vi "TEST_ASIC_MAJ_NEW.vi"(7 "Serial Number":string="SN_1234", 8 "error in":errorcluster, 11 "Instrument VISA in":T1={"AWG VISA"="AgilentGenerator1", "Oscilloscope  VISA "="AgilentOsciloscope", "Integration Board IP"="172.16.17.47", "connection ID"=refnum, "report out"=refnum, "report file path"=path "C:/Users/omartinez/Desktop/L0nL1_Results"}) -> (0 "error out":errorcluster, 3 "Instrument VISA out":T1={"AWG VISA"="AgilentGenerator1", "Oscilloscope  VISA "="AgilentOsciloscope", "Integration Board IP"="172.16.17.47", "connection ID"=refnum, "report out"=refnum, "report file path"=path "C:/Users/omartinez/Desktop/L0nL1_Results"}, 5 "ThresholdOut":i32[][](array[numeric])=[[526, 520, 522, 524, 510, 512, 524]])   [LabVIEW 2012]
uses:
  <vilib>/Utility/NIReport.llb/NI_report.lvclass
  <vilib>/Utility/NIReport.llb/HTML/NI_HTML.lvclass
  <instrlib>/Agilent 8000 Series/Public/Configure/Configure Math (Binary Operation).vi
  Sum_Abrilader/L0_Sum_Adder Folder/C/Program Files/National Instruments/LabVIEW 2012/instr.lib/Agilent 8000 Series/Public/Data/Low Level/Fetch Measurement (More).vi
  <instrlib>/Agilent 8000 Series/Agilent 8000 Series.lvlib
  Sum_Abrilader/L0_Sum_Adder Folder/C/Program Files/National Instruments/LabVIEW 2012/instr.lib/Agilent 81150/Agilent 81150.lvlib
panel:
  in  "Clip_sel_b":u32=1
  in  "Ib_clipVb":u32=63
  in  "Att gain":u32=15
  out "threshold out":i32=524
  in  "Threshold Limits":i32[](array[numeric])=[500, 1024]
  in  "Channels":i32[](array[numeric])=[0, 1, 2, 3, 4, 5, 6]
  in  "Voltages comprobation":dbl[](array[numeric])=[0.05, 0.1, 0.2, 0.5, 0.8]
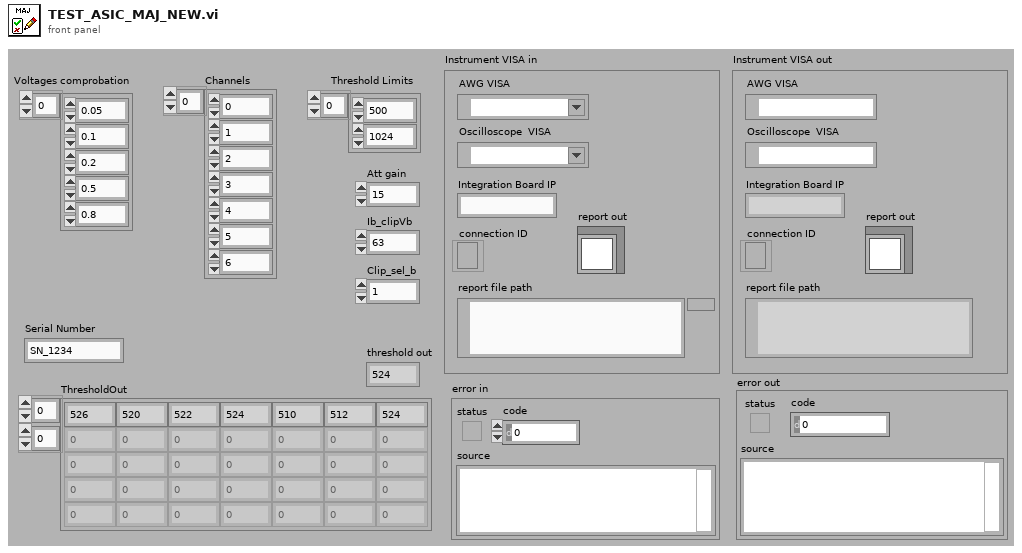
[diagram p1: front panel]
types:
  T1 = cluster{"AWG VISA":refnum<visa-resource-name>, "Oscilloscope  VISA ":refnum<visa-resource-name>, "Integration Board IP":string, "connection ID":refnum<k5>, "report out":refnum<class "NI_report.lvclass">, "report file path":path}
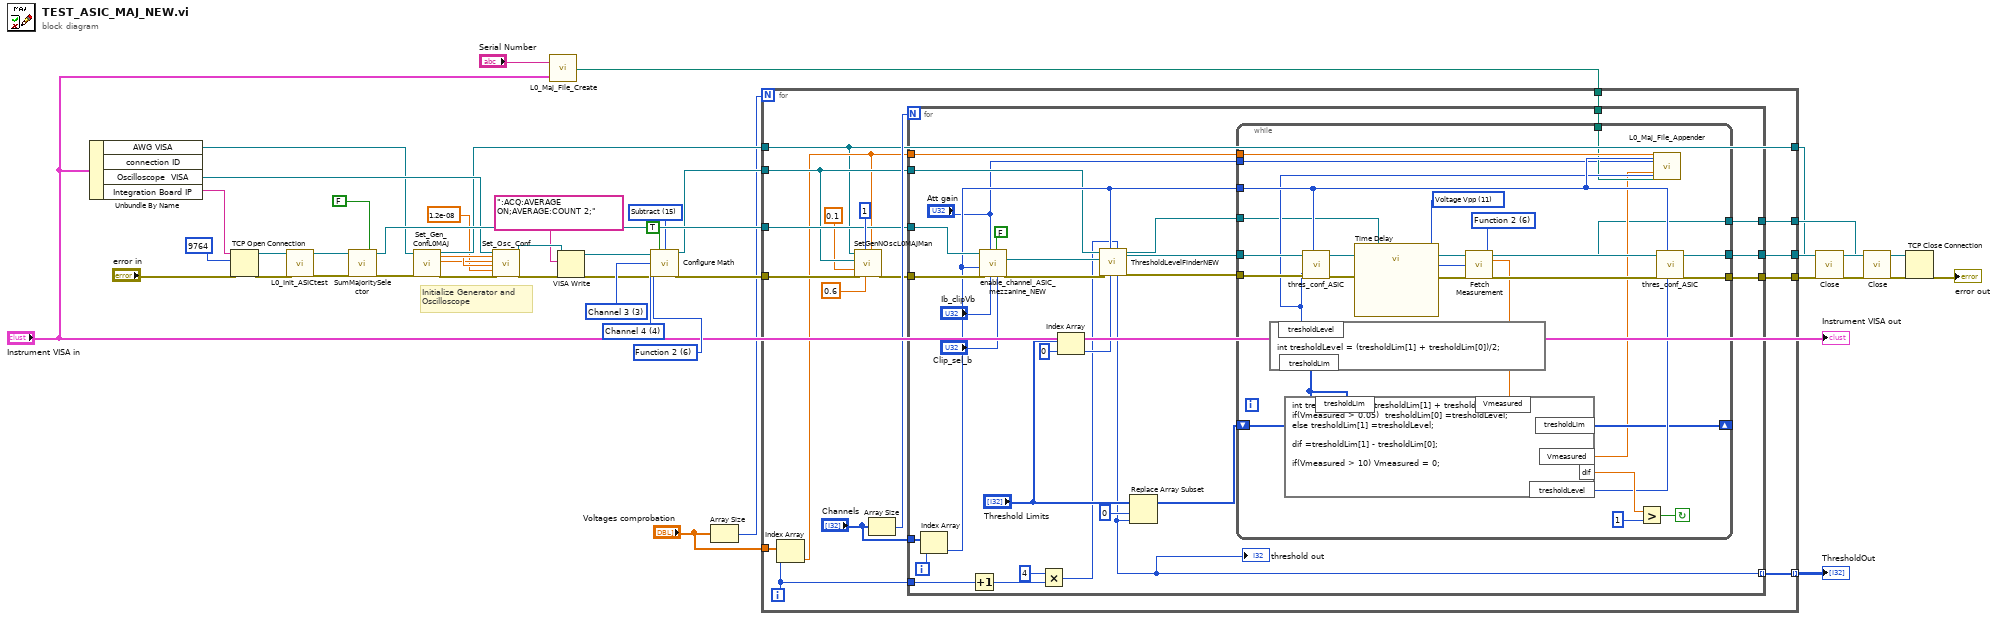
[diagram p0: block diagram]
diagram:
  w30 = u16 6 items=["Function 1"=5, "Function 2"=6, "Function 3"=7, "Function 4"=8] ("Math Channel (5: Function 1)")
  w31 = u16 15 items=["Add"=12, "Divide"=13, "Multiply"=14, "Subtract"=15, "Common Mode"=16, "Versus"=17] ("Math Operation (12: Add)")
  w29 = 3 items=["Channel 1"=1, "Channel 2"=2, "Channel 3"=3, "Channel 4"=4] ("Channel (1: Channel 1)")
  w28 = 4 items=["Channel 1"=1, "Channel 2"=2, "Channel 3"=3, "Channel 4"=4] ("Channel (1: Channel 1)")
  # "Initialize Generator and \nOscilloscope"
  n1 = Unbundle By Name("Instrument VISA in") -> ("AWG VISA"=w7:refnum<visa-resource-name>, "Oscilloscope  VISA"=w11:refnum<visa-resource-name>, "Integration Board IP"=w40:string)  [unwired: 1 out]
  n2 = TCP Open Connection(address=w40, remote port or service name=u16 9764, error in (no error)="error in") -> (connection ID=w34:refnum<k5>, error out=w35:errorcluster)  [unwired: 2 in]
  n3 = call "L0_Init_ASICtest.vi"("error in"=w35, "connection ID in"=w34) -> ("error out"=w36:errorcluster, "connection ID out"=w33:refnum<k5>)  [unwired: 8 in]
  n4 = call "SumMajoritySelector.vi"("On Sum\nOff Majority"=FALSE ("On Sum\nOff Majority"), "error in (no error)"=w36, "connection ID"=w33) -> ("error out"=w8:errorcluster, "connection ID out"=w39:refnum<k5>)  [unwired: 5 in]
  n5 = call "Set_Gen_ConfL0MAJ.vi"("AWG VISA"=w7, "error in (no error)"=w8) -> ("Amplitude 1 OUT"=w16:dbl, "VISA resource name out"=w6:refnum<visa-resource-name>, "Pulse Width in seconds 1 OUT"=w15:dbl, "Trigger Level 1"=w14:dbl, "error out"=w17:errorcluster)  [unwired: 10 in, 3 out]
  n6 = call "Set_Osc_Conf.vi"("VISA resource name"=w11, "Amplitude IN"=w16, "Trigger Level IN"=w14, "Pulse Width in seconds IN"=w15, "Position 1"=1.2e-08, "error in (no error)"=w17) -> ("VISA resource name out"=w12:refnum<visa-resource-name>, "error out"=w13:errorcluster)  [unwired: 12 in]
  n7 = call "L0_Maj_File_Create.vi"("input cluster"="Instrument VISA in", "Serial Number"="Serial Number") -> ("appended path"=w21:path)
  n8 = VISA Write(VISA resource name=w12, write buffer=":ACQ:AVERAGE ON;AVERAGE:COUNT 2;", error in (no error)=w13) -> (VISA resource name out=w10:refnum<visa-resource-name>, error out=w9:errorcluster)  [unwired: 1 out]
  n9 = call-poly <instrlib>:"Configure Math.vi"("VISA resource name"=w10, "Enable Math Channel (T:Enable)"=TRUE, "Math Operation (12: Add)"=w31, "Math Channel (5: Function 1)"=w30, "Math Operand (1: Channel 1)"=w29, "Math Operand (2: Channel 2)"=w28, "error in (no error)"=w9) -> ("VISA resource name out"=w26:refnum<visa-resource-name>, "error out"=w27:errorcluster)  [unwired: 7 in]
  n10 = Array Size(array="Voltages comprobation") -> (size(s)=w1:i32)
  n11 = for {
    N: w1 -> [_]
    tunnel: [w61] -> w19
    tunnel: [w60] -> w41
    tunnel: w27 -> [w56]
    tunnel: w39 -> [w52]
    tunnel: w6 -> [w44]
    tunnel: w26 -> [w51]
    tunnel: "Voltages comprobation" -> [w59]
    tunnel: [w50] -> w24 mode=indexing
    tunnel: w21 -> [w49]
    tunnel: [w45] -> w5
    tunnel: [w44] -> w4
    i -> [w46]
    n12 = Index Array(array=w59, index=w46) -> (element=w47:dbl)
    n13 = call "SetGenNOscL0MAJMan.vi"("Input Voltage"=w47, "Amp Scaler"=0.6, "NChannels"=1, "error in (no error)"=w56, "Output Voltage"=0.1 ("Input Voltage"), "VISA resource name"=w51, "AWG VISA"=w44) -> ("error out 2"=w53:errorcluster)  [unwired: 4 in]
    n14 = Array Size(array="Channels") -> (size(s)=w54:i32)
    n15 = for {
      N: w54 -> [_]
      tunnel: [w90] -> w61
      tunnel: [w89] -> w60
      tunnel: "Channels" -> [w87]
      tunnel: w53 -> [w86]
      tunnel: w52 -> [w82]
      tunnel: w51 -> [w79]
      tunnel: w47 -> [w74]
      tunnel: [w64] -> w50 mode=indexing
      tunnel: w49 -> [w72]
      tunnel: w46 -> [w68]
      tunnel: [w66] -> w45
      i -> [w88]
      n16 = Index Array(array=w87, index=w88) -> (element=w81:i32)
      n17 = Increment(x=w68) -> (x+1=w65:i32)
      n18 = call "enable_channel_ASIC_mezzanine_NEW.vi"("Clip_sel_b"="Clip_sel_b", "maj/sum"=FALSE, "Ib_clipVb"="Ib_clipVb", "Att gain"="Att gain", "error in"=w86, "Channel"=w81, "connection ID"=w82) -> ("error out"=w80:errorcluster, "connection ID out"=w78:refnum<k5>)  [unwired: 2 in, 1 out]
      n19 = Multiply(x=4, y=w65) -> (x*y=w63:i32)
      n20 = Index Array(array="Threshold Limits", index=0) -> (element=w77:i32)
      n21 = call "ThresholdLevelFinderNEW.vi"("correction"=w63, "Initial Threshold"=w77, "Channel"=w81, "error in (no error)"=w80, "connection ID"=w78, "VISA resource name"=w79) -> ("error out"=w62:errorcluster, "connection ID out"=w75:refnum<k5>, "VISA resource name out"=w73:refnum<visa-resource-name>, "threshold out"=w64:i32)  [unwired: 1 in, 1 out]
      "threshold out" <- w64
      n22 = Replace Array Subset(array="Threshold Limits", new element=w64, index=u32 0 ("Att gain")) -> (w76:i32[])
      n23 = while {
        tunnel: [w105] -> w90
        tunnel: [w104] -> w89
        tunnel: w81 -> [w102]
        tunnel: w75 -> [w116]
        tunnel: w62 -> [w115]
        shift-right: [w98] -> _
        shift-left: w76 -> [w111]
        tunnel: w74 -> [w103]
        tunnel: w73 -> [w99]
        tunnel: w72 -> [w97]
        tunnel: "Att gain" -> [w94]
        tunnel: [w93] -> w66
        stop <- w112 continue-if-true
        w109 = 11 items=["Rise Time", "Fall Time", "Frequency", "Period", "Voltage RMS(AC)", "Voltage RMS(DC)", "Voltage RMS (AC,cycle)", "Voltage RMS (DC,cycle)", "Voltage Max", "Voltage Min", "Voltage Middle", "Voltage Vpp", "Voltage High", "Voltage Low", "Voltage Average", "Voltage Average (cycle)", "Width Negative", "Width Positive", "Duty Cycle Positive", "Amplitude", "Overshoot", "Preshoot", "Voltage Base", "Voltage Upper", "Time Max", "Time Min", "Color Grade Crossing", "Color Grade Eye Width", "Color Grade Eye Height", "Color Grade Eye Q-Factory", "Color Grade Eye Duty Cycle Distortion(Percent)", "Color Grade Eye Duty Cycle Distortion(Time)", "Color Grade Eye Jitter(PP)", "Color Grade Eye Width(RMS)", "Cycle-cycle Duty Jitter(Rising)", "Cycle-cycle Duty Jitter(Falling)", "Cycle-cycle Jitter(Rising)", "Cycle-cycle Jitter(Falling)", "Cycle-cycle - Width", "Cycle-cycle + Width", "Date Rate", "Unit Interval", "FFT Delta Frequency", "FFT Delta Magnitude", "FFT Frequency", "FFT Magnitude", "Slew Rate", "Area (Entire Display)", "Area(Single Cycle)", "Duty Cycle (Rising)", "Duty Cycle (Falling)"] ("Measurement Function (0: Rise Time)")
        w110 = 6 items=["Channel 1"=1, "Channel 2"=2, "Channel 3"=3, "Channel 4"=4, "Function 1"=5, "Function 2"=6, "Function 3"=7, "Function 4"=8, "Memory 1"=9, "Memory 2"=10, "Memory 3"=11, "Memory 4"=12] ("Channel (1: Channel 1)")
        n24 = formula code="int tresholdLevel = (tresholdLim[1] + tresholdLim[0])/2;"("tresholdLim"=w111) -> ("tresholdLevel"=w101:i32)
        n25 = call "thres_conf_ASIC.vi"("threshold"=w101, "Ring"=w102, "error out 3"=w115, "connection ID"=w116) -> ("error out 2"=w108:errorcluster, "connection ID out"=w106:refnum<k5>)  [unwired: 4 in, 2 out]
        n26 = call "Time Delay"("error in (no error)"=w108) -> ("error out"=w92:errorcluster)  [unwired: 10 in]
        n27 = call-poly "Fetch Measurement.vi"("VISA resource name"=w99, "Channel (1: Channel 1)"=w110, "Measurement Function (0: Rise Time)"=w109, "error in (no error)"=w92) -> ("VISA resource name out"=w93:refnum<visa-resource-name>, "Measurement"=w96:dbl, "error out"=w107:errorcluster)  [unwired: 9 in]
        n28 = formula code="int tresholdLevel = (tresholdLim[1] + tresholdLim[0])/2;\nif(Vmeasured > 0.05)  tresholdLim[0] =tresholdLevel;\nelse tresholdLim[1] =tresholdLevel;\n\ndif =tresholdLim[1] - tresholdLim[0];\n\nif(Vmeasured > 10) Vmeasured = 0;"("Vmeasured"=w96, "tresholdLim"=w111) -> ("dif"=w113:dbl, "tresholdLevel"=w100:i32, "tresholdLim"=w98:i32[], "Vmeasured"=w95:dbl)
        n29 = Greater?(x=w113, y=1) -> (0:w112:bool)
        n30 = call "L0_Maj_File_Appender.vi"("Vin"=w103, "CH"=w102, "Att"=w94, "Vmeas"=w95, "Threshold"=w101, "file path (dialog if empty)"=w97) -> ()  [unwired: 22 in]
        n31 = call "thres_conf_ASIC.vi"("threshold"=w100, "Ring"=w102, "error out 3"=w107, "connection ID"=w106) -> ("error out 2"=w105:errorcluster, "connection ID out"=w104:refnum<k5>)  [unwired: 4 in, 2 out]
      }
    }
  }
  "ThresholdOut" <- w24
  n32 = call <instrlib>:"Close.vi"("error in (no error)"=w19, "VISA resource name"=w4) -> ("error out"=w20:errorcluster)  [unwired: 9 in]
  n33 = call <instrlib>:"Close.vi"("error in (no error)"=w20, "VISA resource name"=w5) -> ("error out"=w18:errorcluster)  [unwired: 9 in]
  n34 = TCP Close Connection(connection ID=w41, error in (no error)=w18) -> (error out=→"error out":errorcluster)  [unwired: 1 in, 1 out]
  "Instrument VISA out" <- "Instrument VISA in"
